vi "setSerializedData.vi"(0 "reference":refnum<class "InitialStateNode.lvclass">, 1 "parent":refnum<class "AbstractNode.lvclass">, 2 "children":refnum<class "AbstractNode.lvclass">[](array[class]), 3 "xmlOut":string, 5 "error in (no error)":errorcluster) -> (14 "reference out":refnum<class "InitialStateNode.lvclass">, 19 "error out":errorcluster)   [LabVIEW 2014, in "InitialStateNode.lvclass"]
doc: "setSerializedData"
uses:
  <resource>/Framework/Providers/Open_GDS/UML/InitialStateNode_class/InitialStateNode.lvclass
  <resource>/Framework/Providers/Open_GDS/UML/AbstractNode_class/AbstractNode.lvclass
  <resource>/Framework/Providers/Open_GDS/UML/AbstractNode_class/ObjectReference.ctl
  <resource>/Framework/Providers/Open_GDS/UML/General/Rectangle/Rectangle Rectangle2D.ctl
  <resource>/Framework/Providers/Open_GDS/UML/MultiLineString_class/ObjectReference.ctl
  <resource>/Framework/Providers/Open_GDS/UML/MultiLineString_class/MultiLineString.lvclass
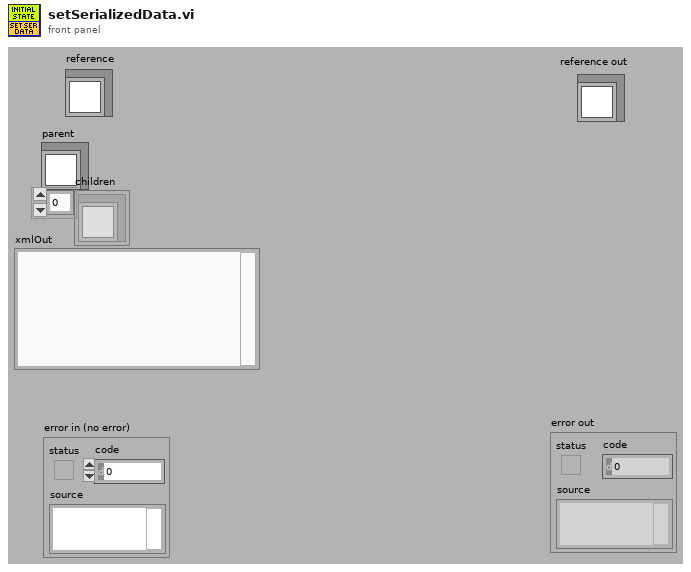
[diagram p1: front panel]
types:
  T1 = typedef "AbstractNode.lvclass/ObjectReference.ctl" = refnum<k1>
  T2 = typedef "Rectangle Rectangle2D.ctl" = cluster{"x":dbl, "y":dbl, "width":dbl, "height":dbl}
  T3 = typedef "MultiLineString.lvclass/ObjectReference.ctl" = refnum<k1>
  T4 = cluster{"Base class":cluster{"Base class":cluster{"parent":T1, "children":T1[]}, "bounds":T2}, "name":T3, "DEFAULT_WIDTH":i32, "DEFAULT_HEIGHT":i32}
  T5 = typedef "InitialStateNode.lvclass/ObjectAttributes.ctl" = cluster{"Base class":T6, "name":refnum<class "MultiLineString.lvclass">, "DEFAULT_WIDTH":i32, "DEFAULT_HEIGHT":i32}
  T6 = typedef "RectangularNode.lvclass/ObjectAttributes.ctl" = cluster{"Base class":T7, "bounds":T2}
  T7 = typedef "AbstractNode.lvclass/ObjectAttributes.ctl" = cluster{"parent":refnum<class "AbstractNode.lvclass">, "children":refnum<class "AbstractNode.lvclass">[], "Hidden":bool}
  T8 = cluster{"Attributes":cluster{"Base class":cluster{"Base class":cluster{"parent":T1, "children":T1[]}, "bounds":T2}, "name":T3, "DEFAULT_WIDTH":i32, "DEFAULT_HEIGHT":i32}, string}
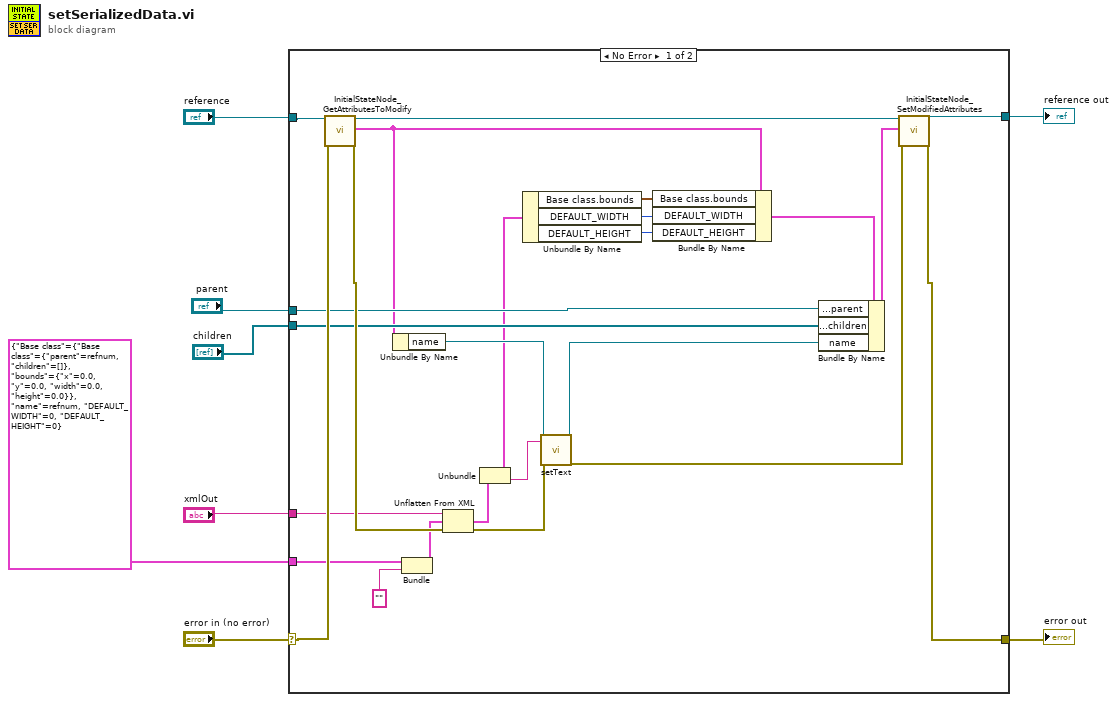
[diagram p0: block diagram]
diagram:
  n1 = case shown="No Error" "error in (no error)" {
    selector: "error in (no error)" -> [w23 w34]
    tunnel: "reference" -> [w24 w35]
    tunnel: [w22 w34] -> w6
    tunnel: [w20 w35] -> w5
    tunnel: "xmlOut" -> [w21 _]
    tunnel: "parent" -> [w19 _]
    tunnel: "children" -> [w18 _]
    tunnel: T4 {"Base class"={"Base class"={"parent"=refnum, "children"=[]}, "bounds"={"x"=0.0, "y"=0.0, "width"=0.0, "height"=0.0}}, "name"=refnum, "DEFAULT_WIDTH"=0, "DEFAULT_HEIGHT"=0} ("Attributes") -> [w15 _]
    frame No Error {
      n2 = call <resource>:"InitialStateNode_GetAttributesToModify.vi"("reference in"=w24, "error in (no error)"=w23) -> ("reference out"=w33:refnum<class "InitialStateNode.lvclass">, "Attributes"=w10:T5, "error out"=w31:errorcluster)  [unwired: 1 in, 14 out]
      n3 = Unbundle By Name(w10) -> ("name"=w30:refnum<class "MultiLineString.lvclass">)
      n4 = Bundle("Attributes"=w15, "") -> (w29:T8)  [unwired: 1 out]
      n5 = Unflatten From XML(xml string=w21, type=w29, error in (no error)=w31) -> (value=w26:T8, error out=w28:errorcluster)
      n6 = Unbundle(w26) -> ("Attributes"=w11:T4, w25:string)
      n7 = Unbundle By Name(w11) -> ("Base class.bounds"=w14:T2, "DEFAULT_WIDTH"=w13:i32, "DEFAULT_HEIGHT"=w12:i32)
      n8 = call-dynamic "setText.vi"("reference"=w30, "text"=w25, "error in (no error)"=w28) -> ("reference out"=w27:refnum<class "MultiLineString.lvclass">, "error out"=w16:errorcluster)  [unwired: 15 out]
      n9 = Bundle By Name(cluster=w10, "Base class.bounds"=w14, "DEFAULT_WIDTH"=w13, "DEFAULT_HEIGHT"=w12) -> (w9:T5)
      n10 = Bundle By Name(cluster=w9, "Base class.Base class.parent"=w19, "Base class.Base class.children"=w18, "name"=w27) -> (w32:T5)
      n11 = call <resource>:"InitialStateNode_SetModifiedAttributes.vi"("reference in"=w33, "Attributes"=w32, "error in (no error)"=w16) -> ("reference out"=w20:refnum<class "InitialStateNode.lvclass">, "error out"=w22:errorcluster)  [unwired: 3 in, 12 out]
    }
    frame Error {
    }
  }
  "reference out" <- w5
  "error out" <- w6
